vi "HapticSTM.vi"() -> ()   [LabVIEW 2017]
uses:
  <userlib>/PositionDLL/PositionDLL.lvlib
panel:
  out "Target Z":dbl
  out "Target X":dbl
  out "Z Out":dbl
  out "X Out":dbl
  out "Max speed":dbl
  out "FW":dbl
  out "VY":dbl
  out "VZ":dbl
  out "VX":dbl
  in  "Drag":dbl=1.0
  in  "STOP":bool
  in  "START":bool
  out "Fy":dbl
  out "Fz":dbl
  out "phi":dbl
  out "psi":dbl
  out "Fx":dbl
  out "theta":dbl
  out "x":dbl
  out "y":dbl
  out "z":dbl
  in  "Sensitivity":dbl=3.5
  out "Clicks":dbl
  out "Scope":dbl
  out "FH":dbl
  out "XI":dbl
  out "ZI":dbl
  # "Sample Window"
  # "Position"
  # "Force"
  # "Angles"
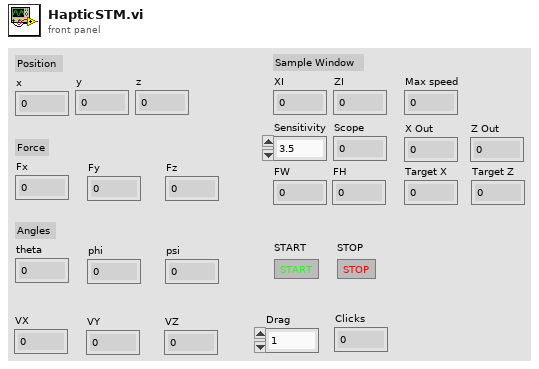
[diagram p1: front panel]
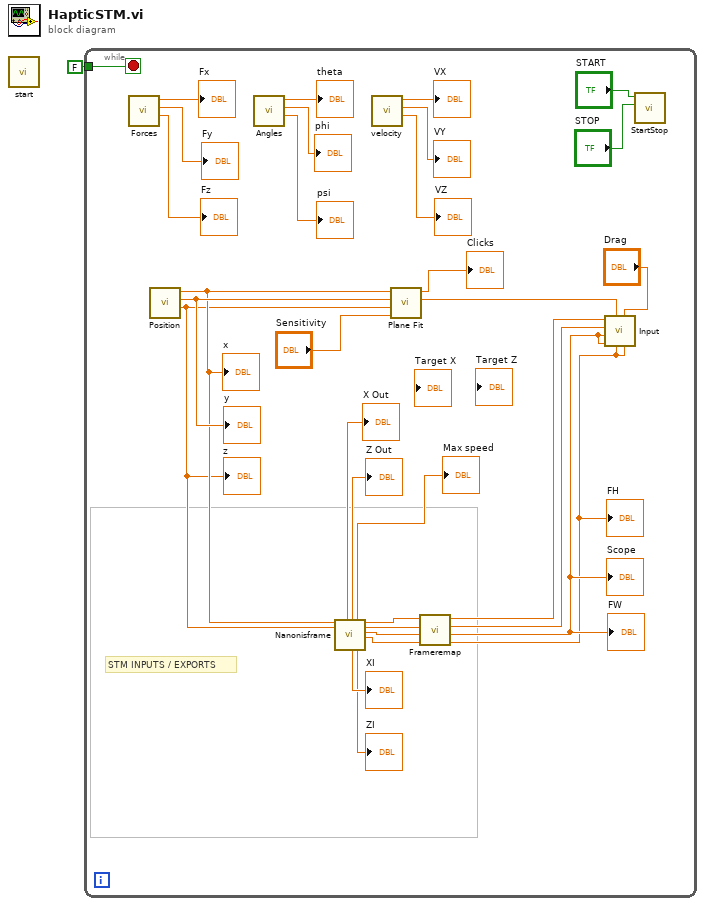
[diagram p0: block diagram]
diagram:
  n1 = call <userlib>:"start.vi"() -> ()  [unwired: 11 in, 1 out]
  n2 = while {
    tunnel: FALSE -> [w21]
    stop <- w21 stop-if-true
    # "STM INPUTS / EXPORTS"
    n3 = call "Forces.vi"() -> ("Fz"=→"Fz":dbl, "Fy"=→"Fy":dbl, "Fx"=→"Fx":dbl)  [unwired: 9 in]
    n4 = call "Position.vi"() -> ("Z"=w10:dbl, "Y"=w28:dbl, "X"=w11:dbl)  [unwired: 9 in]
    "x" <- w11
    "y" <- w28
    "z" <- w10
    n5 = call "Angles.vi"() -> ("psi"=→"psi":dbl, "phi"=→"phi":dbl, "theta"=→"theta":dbl)  [unwired: 9 in]
    n6 = call "Nanonisframe.vi"("x"=w11, "z"=w10) -> ("X Out"=→"X Out":dbl, "Z Out"=→"Z Out":dbl, "Target X"=→"XI":dbl, "Speed"=→"Max speed":dbl, "Target Z"=→"ZI":dbl, "FO X"=w9:dbl, "FO Z"=w8:dbl, "FW"=w7:dbl, "FH"=w6:dbl)  [unwired: 9 in]
    n7 = call "velocity.vi"() -> ("VZ"=→"VZ":dbl, "VY"=→"VY":dbl, "VX"=→"VX":dbl)  [unwired: 9 in]
    n8 = call "Plane Fit.vi"("Sensitivity"="Sensitivity", "Z"=w10, "Y"=w28, "X"=w11) -> ("Output"=w25:dbl, "Clicks"=→"Clicks":dbl)  [unwired: 6 in]
    n9 = call <userlib>:"Frameremap.vi"("FH"=w6, "FW"=w7, "FO Z"=w8, "FO X"=w9) -> ("FH"=w13:dbl, "FW"=w14:dbl, "Z Origin"=w23:dbl, "X Origin"=w24:dbl)  [unwired: 4 in]
    "Scope" <- w14
    "FH" <- w13
    "FW" <- w14
    n10 = call "Input.vi"("Scopez"=w13, "Drag"="Drag", "FH"=w13, "Signal in"=w25, "FW"=w14, "Scopex"=w14, "Z origin"=w23, "X origin"=w24) -> ()  [unwired: 4 in]
    n11 = call "StartStop.vi"("STOP"="STOP", "START"="START") -> ()  [unwired: 10 in]
  }
